vi "Dialog TDMS Datalog.vi"(8 "Error In":errorcluster, 11 "Logdata":string[][](array[string])) -> (0 "Error Out":errorcluster)   [LabVIEW 2019, in "GUI.lvlib"]
uses:
  GUI.lvlib
  <vilib>/Utility/miscctls.llb/LVRowAndColumnUnsignedTypeDef.ctl
  Controls/WebDAV states.ctl
panel:
  in  "Delete":bool
  in  "TDMS List":i32[](listbox)
  in  "Download":bool
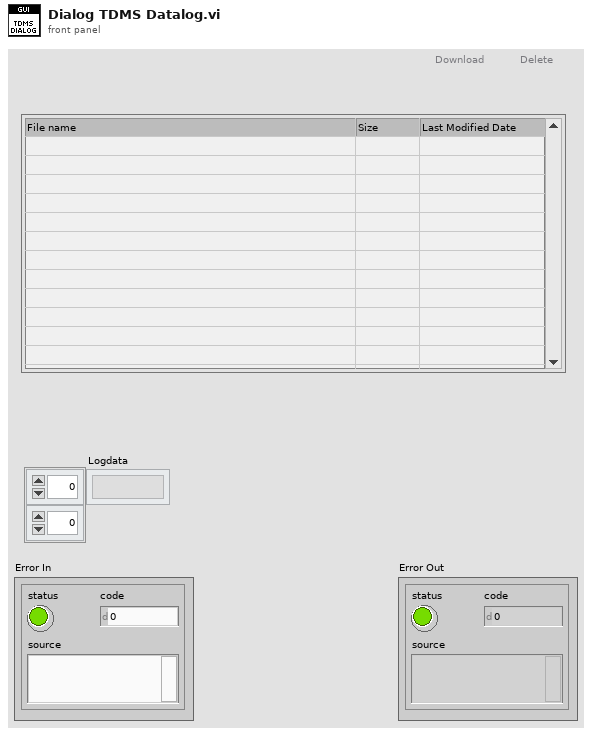
[diagram p1: front panel]
types:
  T1 = typedef "LVRowAndColumnUnsignedTypeDef.ctl" = cluster{"Row":u32, "Column":u32}
  T2 = typedef "GUI.lvlib/WebDAV states.ctl" = enum16{"Open Sess", "Refresh Dir", "Create Dir", "Upload", "Download", "Delete", "Close Sess"}
  T3 = typedef "NI_WebDAV.lvlib/FileInfo.ctl" = cluster{"type":string, "size":u64, "last modification":timestamp, "display name":string, "uri":string}
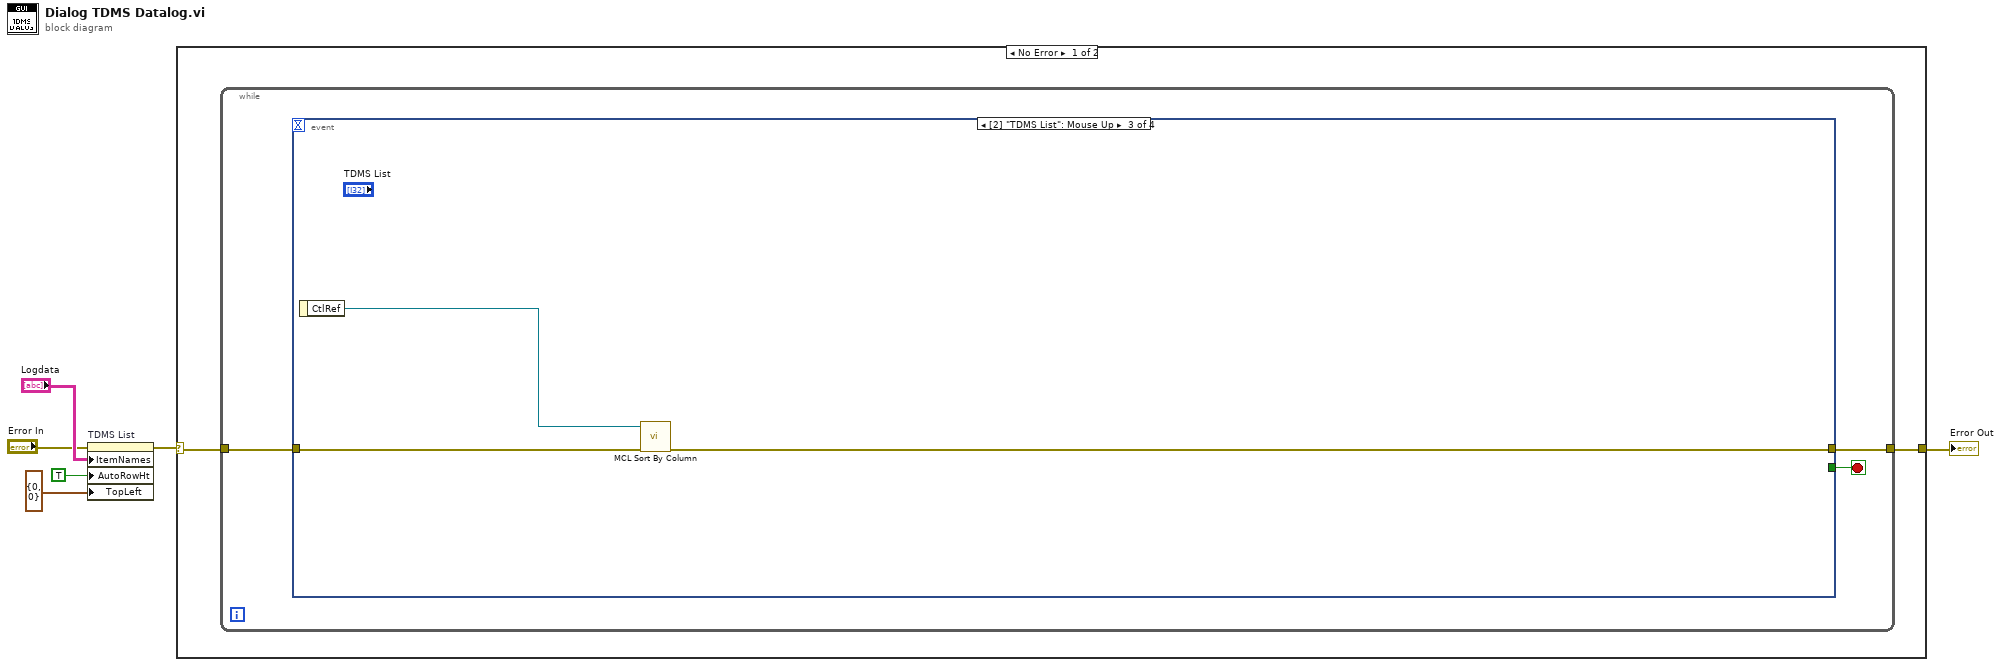
[diagram p0: block diagram]
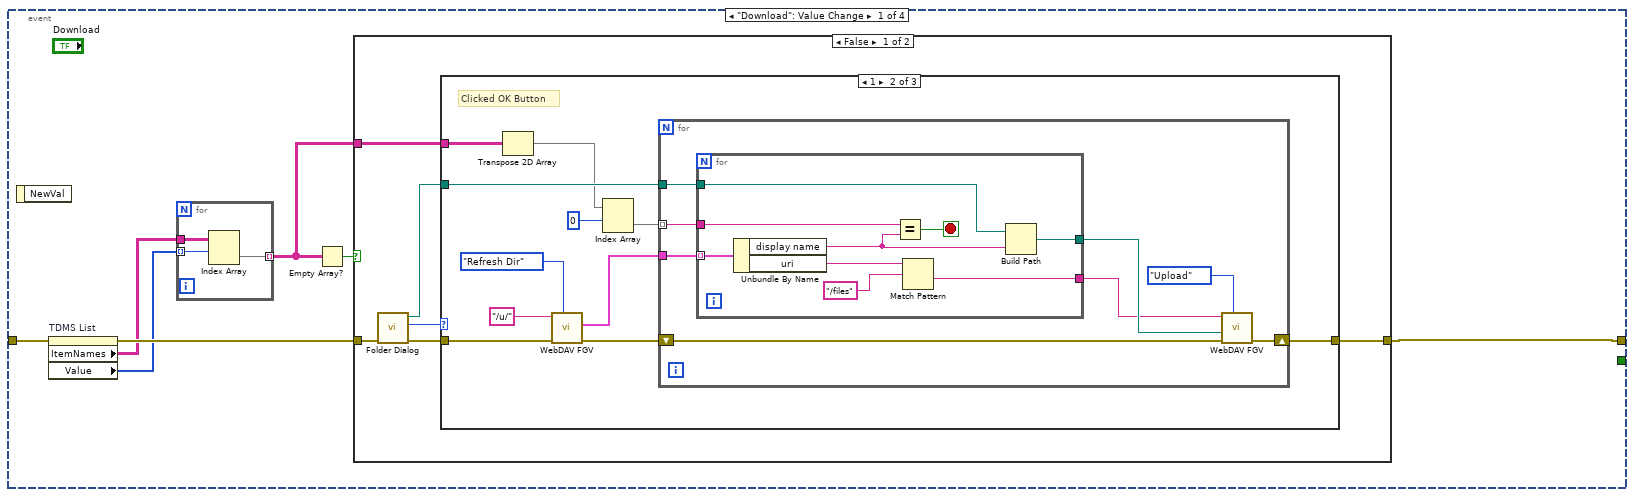
[diagram p2: hidden frame]
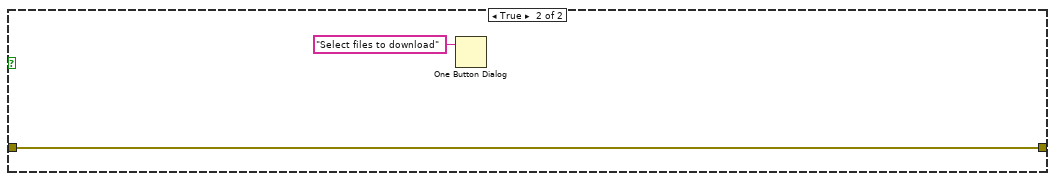
[diagram p5: hidden frame]
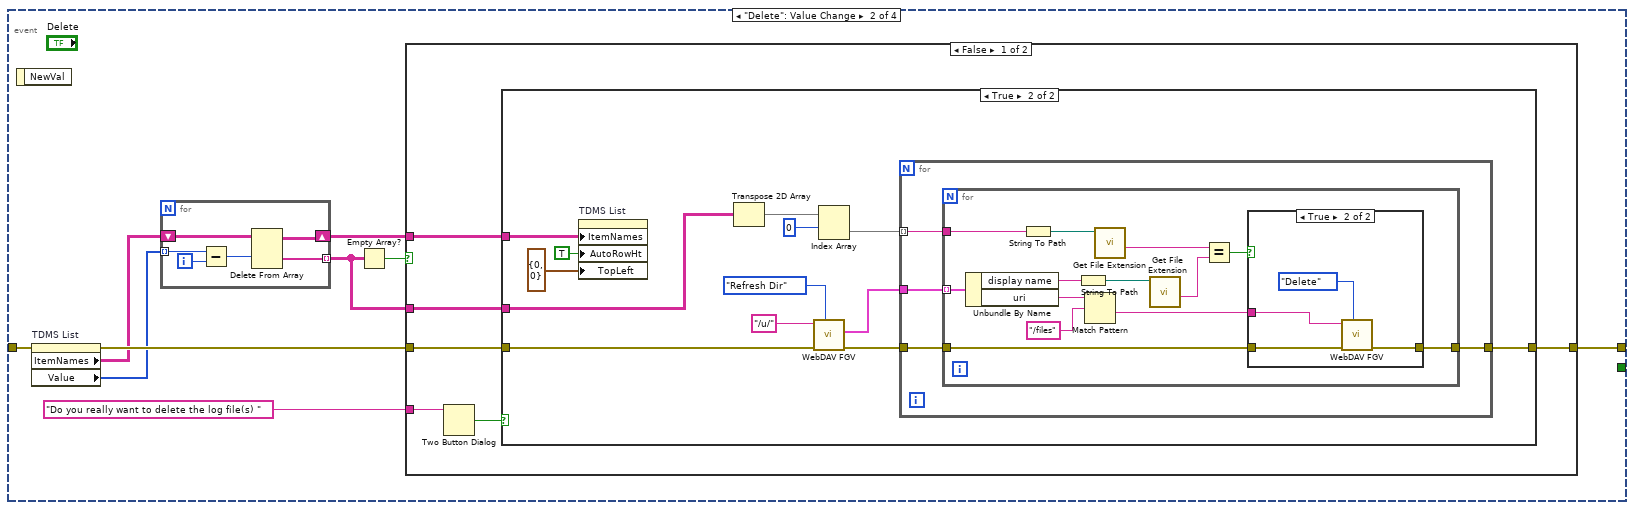
[diagram p6: hidden frame]
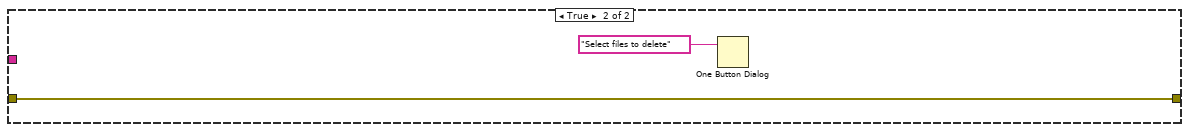
[diagram p9: hidden frame]
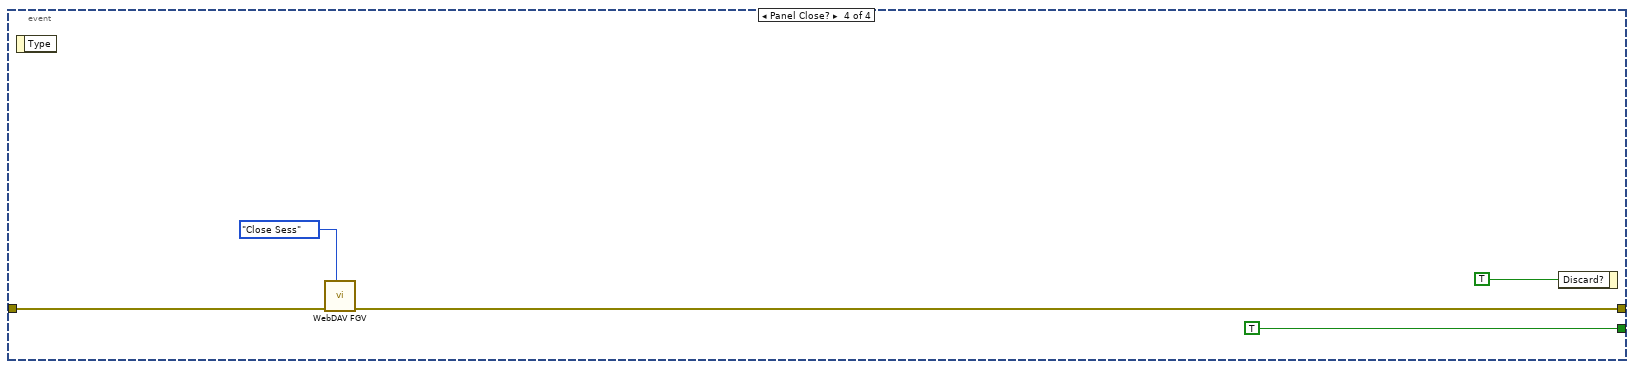
[diagram p10: hidden frame]
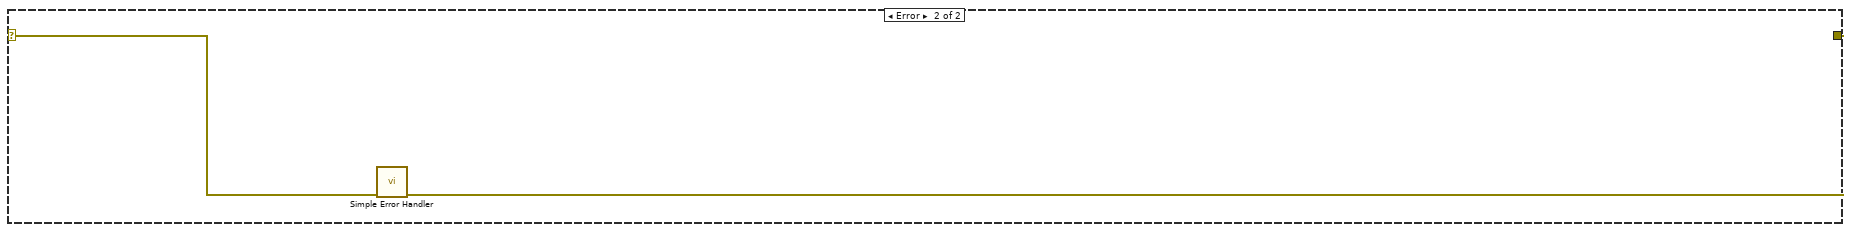
[diagram p11: hidden frame]
diagram:
  n1 = property on="TDMS List" class="MCListbox (strict)"(error in="Error In", "ItemNames"="Logdata", "AutoRowHt"=TRUE ("Autosizing Row Height"), "TopLeft"=T1 {"Row"=0, "Column"=0} ("Top Left Visible Cell")) -> (error out=w3:errorcluster)  [unwired: 1 in, 1 out]
  n2 = case shown="No Error" w3 {
    selector: w3 -> [w7 w128]
    tunnel: [w8 w127] -> w6
    frame No Error {
      n3 = while {
        tunnel: w7 -> [w10]
        tunnel: [w9] -> w8
        stop <- w11 stop-if-true
        n4 = event shown="[2] \"TDMS List\": Mouse Up" {
          selector: _ -> [_ _ _ _]
          dyn-events: _ -> [_ _ _ _]
          timeout: _ -> [_ _ _ _]
          tunnel: [_ _ _ TRUE] -> w11
          tunnel: w10 -> [w16 w65 w121 w123]
          tunnel: [w12 w67 w120 w122] -> w9
          event "Download": Value Change {
            n5 = event-data() -> ()  [unwired: 1 in, 1 out]
            n6 = property on="TDMS List" class="MCListbox (strict)"(error in=w16) -> (error out=w15:errorcluster, "ItemNames"=w14:string[][], "Value"=w13:i32[])  [unwired: 1 in, 1 out]
            n7 = for {
              tunnel: w14 -> [w59]
              tunnel: [w58] -> w17 mode=indexing
              tunnel: w13 -> [w57] mode=indexing
              n8 = Index Array(array=w59, index (row)=w57) -> (element=w58:string[])  [unwired: 1 in]
            }
            n9 = Empty Array?(array=w17) -> (empty?=w18:bool)
            n10 = case shown="False" w18 {
              tunnel: w15 -> [w24 w55]
              tunnel: w17 -> [w19 _]
              tunnel: [w20 w55] -> w12
              frame False {
                n11 = call "Folder Dialog.vi"("error in"=w24) -> ("error out"=w21:errorcluster, "ButtonPressed"=w22:i32, "Path"=w23:path)  [unwired: 8 in]
                n12 = case shown="1" w22 {
                  tunnel: w23 -> [_ w30 _]
                  tunnel: w21 -> [w25 w35 w54]
                  tunnel: [w25 w32 w54] -> w20
                  tunnel: w19 -> [_ w29 _]
                  frame 0, Default {
                    # "None Button Pressed"
                  }
                  frame 1 {
                    # "Clicked OK Button"
                    n13 = Transpose 2D Array(2D array=w29) -> (transposed array=w28:string[][])
                    n14 = call "WebDAV FGV.vi"("WebDAV States"=WebDAV_states."Refresh Dir", "error in (no error)"=w35, "relative uri"="/u/" ("username")) -> ("error out"=w33:errorcluster, "file list"=w31:T3[])  [unwired: 6 in, 1 out]
                    n15 = Index Array(array=w28, index (row)=0) -> (element=w26:string[])  [unwired: 1 in]
                    n16 = for {
                      tunnel: w31 -> [w42]
                      tunnel: w30 -> [w41]
                      tunnel: w26 -> [w37] mode=indexing
                      shift-right: [w43] -> w32
                      shift-left: w33 -> [w44]
                      n17 = for {
                        tunnel: w42 -> [w53] mode=indexing
                        tunnel: w41 -> [w52]
                        tunnel: w37 -> [w51]
                        tunnel: [w49] -> w40
                        tunnel: [w45] -> w39
                        stop <- w50 stop-if-true
                        n18 = Unbundle By Name(w53) -> ("display name"=w48:string, "uri"=w47:string)
                        n19 = Equal?(x=w51, y=w48) -> (x = y?=w50:bool)
                        n20 = Match Pattern(string=w47, regular expression="/files" ("search string/char (-)")) -> (after substring=w45:string)  [unwired: 1 in, 3 out]
                        n21 = Build Path(base path=w52, name or relative path=w48) -> (appended path=w49:path)
                      }
                      n22 = call "WebDAV FGV.vi"("WebDAV States"=WebDAV_states."Upload", "error in (no error)"=w44, "local file path"=w40, "relative uri"=w39) -> ("error out"=w43:errorcluster)  [unwired: 5 in, 2 out]
                    }
                  }
                  frame 2 {
                    # "Clicked Cancel Button"
                  }
                }
              }
              frame True {
                n23 = One Button Dialog(message="Select files to download") -> ()  [unwired: 1 in, 1 out]
              }
            }
          }
          event "Delete": Value Change {
            n24 = event-data() -> ()  [unwired: 1 in, 1 out]
            n25 = property on="TDMS List" class="MCListbox (strict)"(error in=w65) -> (error out=w64:errorcluster, "ItemNames"=w63:string[][], "Value"=w62:i32[])  [unwired: 1 in, 1 out]
            n26 = for {
              tunnel: w62 -> [w113] mode=indexing
              shift-right: [w115] -> w60
              shift-left: w63 -> [w117]
              tunnel: [w114] -> w61 mode=indexing
              i -> [w118]
              n27 = Subtract(x=w113, y=w118) -> (x-y=w116:i32)
              n28 = Delete From Array(array=w117, index (row)=w116) -> (deleted portion=w114:string[], array with subset deleted=w115:string[][])  [unwired: 2 in]
            }
            n29 = Empty Array?(array=w61) -> (empty?=w68:bool)
            n30 = case shown="False" w68 {
              tunnel: w61 -> [w74 _]
              tunnel: w64 -> [w73 w111]
              tunnel: [w72 w111] -> w67
              tunnel: "Do you really want to delete the log file(s) " ("message") -> [w70 _]
              tunnel: w60 -> [w69 _]
              frame False {
                n31 = Two Button Dialog(message=w70) -> (T button?=w71:bool)  [unwired: 2 in]
                n32 = case shown="True" w71 {
                  tunnel: w74 -> [_ w78]
                  tunnel: w73 -> [w75 w76]
                  tunnel: [w75 w81] -> w72
                  tunnel: w69 -> [_ w77]
                  frame False {
                  }
                  frame True {
                    n33 = property on="TDMS List" class="MCListbox (strict)"("ItemNames"=w77, "AutoRowHt"=TRUE ("Autosizing Row Height"), "TopLeft"=T1 {"Row"=0, "Column"=0} ("Top Left Visible Cell")) -> ()  [unwired: 2 in, 2 out]
                    n34 = Transpose 2D Array(2D array=w78) -> (transposed array=w88:string[][])
                    n35 = call "WebDAV FGV.vi"("WebDAV States"=WebDAV_states."Refresh Dir", "error in (no error)"=w76, "relative uri"="/u/" ("username")) -> ("error out"=w84:errorcluster, "file list"=w83:T3[])  [unwired: 6 in, 1 out]
                    n36 = Index Array(array=w88, index (row)=0) -> (element=w82:string[])  [unwired: 1 in]
                    n37 = for {
                      tunnel: w83 -> [w92]
                      tunnel: w82 -> [w91] mode=indexing
                      tunnel: w84 -> [w90]
                      tunnel: [w89] -> w81
                      n38 = for {
                        tunnel: w92 -> [w105] mode=indexing
                        tunnel: w91 -> [w95]
                        tunnel: w90 -> [w99]
                        tunnel: [w96] -> w89
                        n39 = Unbundle By Name(w105) -> ("display name"=w101:string, "uri"=w104:string)
                        n40 = String To Path(string=w95) -> (path=w94:path)
                        n41 = String To Path(string=w101) -> (path=w102:path)
                        n42 = Match Pattern(string=w104, regular expression="/files" ("search string/char (-)")) -> (after substring=w97:string)  [unwired: 1 in, 3 out]
                        n43 = call <vilib>:"Get File Extension.vi"("file"=w94) -> ("filename without extension"=w93:string)  [unwired: 6 in, 4 out]
                        n44 = call <vilib>:"Get File Extension.vi"("file"=w102) -> ("filename without extension"=w100:string)  [unwired: 6 in, 4 out]
                        n45 = Equal?(x=w93, y=w100) -> (x = y?=w98:bool)
                        n46 = case shown="True" w98 {
                          tunnel: w99 -> [w106 w109]
                          tunnel: w97 -> [_ w108]
                          tunnel: [w106 w107] -> w96
                          frame False {
                          }
                          frame True {
                            n47 = call "WebDAV FGV.vi"("WebDAV States"=WebDAV_states."Delete", "error in (no error)"=w109, "relative uri"=w108) -> ("error out"=w107:errorcluster)  [unwired: 6 in, 2 out]
                          }
                        }
                      }
                    }
                  }
                }
              }
              frame True {
                n48 = One Button Dialog(message="Select files to delete") -> ()  [unwired: 1 in, 1 out]
              }
            }
          }
          event "TDMS List": Mouse Up {
            n49 = event-data() -> ("CtlRef"=w119:refnum<vi>)  [unwired: 1 in]
            n50 = call "MCL Sort By Column.vi"("error in (no error)"=w121, "CtlRef"=w119) -> ("error out"=w120:errorcluster)  [unwired: 8 in, 1 out]
          }
          event Panel Close? {
            n51 = event-data() -> ()  [unwired: 1 in, 1 out]
            n52 = call "WebDAV FGV.vi"("WebDAV States"=WebDAV_states."Close Sess", "error in (no error)"=w123) -> ("error out"=w122:errorcluster)  [unwired: 7 in, 2 out]
            n53 = event-data("Discard?"=TRUE) -> ()  [unwired: 1 in, 1 out]
          }
        }
      }
    }
    frame Error {
      n54 = call <vilib>:"Simple Error Handler.vi"("error in (no error)"=w128) -> ("error out"=w127:errorcluster)  [unwired: 4 in, 4 out]
    }
  }
  "Error Out" <- w6
